vi "Chart[Template].TestLauncher.vi"() -> ()   [LabVIEW 2018, in "DisplayWaveform.lvlib" / "DisplayWaveforms.lvclass"]
doc: "JKI State Machine Objects (SMO) 1.0.0.5\nJKI - JKI\nCopyright (c) 2016, JKI"
uses:
  DisplayWaveforms.lvclass
  <vilib>/JKI/JKI SMO/SMO/SMO.lvclass
  <vilib>/JKI/JKI SMO/SMO.UI/SMO.UI.lvclass
  Typedefs/Dependencies--Cluster.ctl
  <vilib>/JKI/JKI SMO/SMO/Typedefs/SMOState --Enum.ctl
  C:/Program Files (x86)/National Instruments/LabVIEW 2020/vi.lib/JKI/JKI SMO/SMO.UI/SMO.UI.lvclass
  C:/Program Files (x86)/National Instruments/LabVIEW 2020/vi.lib/JKI/JKI SMO/SMO/SMO.lvclass
panel:
  in  "Send":bool
  out "error out":errorcluster
  in  "Stop":bool
  # "Chart Test Launcher"
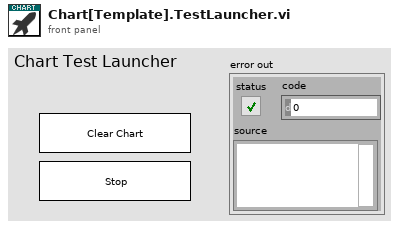
[diagram p1: front panel]
types:
  T1 = typedef "DisplayWaveform.lvlib/DisplayWaveforms.lvclass/Dependencies--Cluster.ctl" = cluster{"New Value":refnum<user-event>}
  T2 = typedef "SMO.lvclass/Public Events.ctl" = cluster{"Error":refnum<user-event>, "State":refnum<user-event>, "Reserve State":refnum<user-event>}
  T3 = typedef "SMO.UI.lvclass/PublicEvents--Cluster.ctl" = cluster{"UI Hidden":refnum<user-event>, "UI State":refnum<user-event>}
  T4 = typedef "DisplayWaveform.lvlib/DisplayWaveforms.lvclass/PublicEvents--Cluster.ctl" = cluster{"Chart Cleared":refnum<user-event>, "Chart Exported":refnum<user-event>, "ChartParams Set":refnum<user-event>}
  T5 = typedef "SMO.lvclass/SMOState --Enum.ctl" = enum16{"unknown", "Created", "Started", "Stopped"}
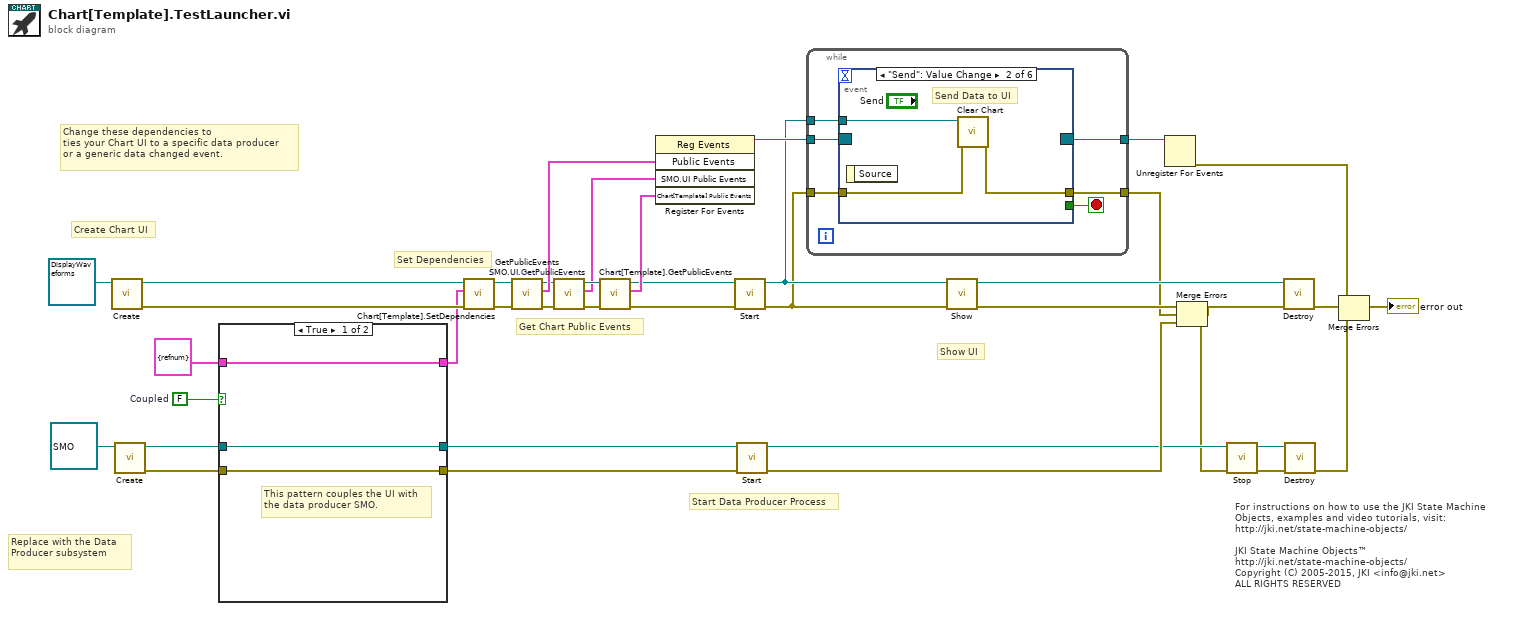
[diagram p0: block diagram]
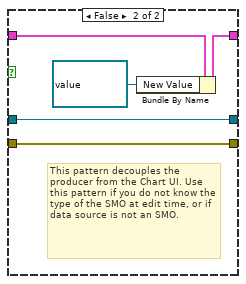
[diagram p2: hidden frame]
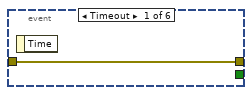
[diagram p3: hidden frame]
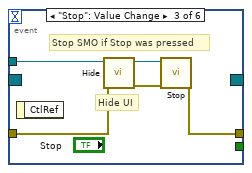
[diagram p4: hidden frame]
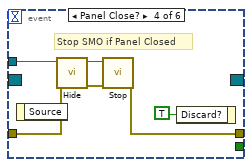
[diagram p5: hidden frame]
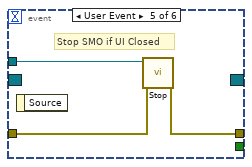
[diagram p6: hidden frame]
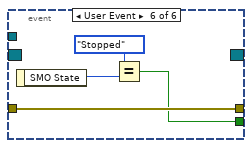
[diagram p7: hidden frame]
diagram:
  w22 = FALSE  # Coupled
  # "Start Data Producer Process"
  # "Set Dependencies"
  # "Create Chart UI"
  # "Replace with the Data Producer subsystem"
  # "Change these dependencies to\nties your Chart UI to a specific data producer\nor a generic data changed event."
  # "Show UI"
  # "For instructions on how to use the JKI State Machine Objects, examples and video tutorials, visit:\nhttp://jki.net/state-machine-objects/\n\nJKI State Machine Objects™\nhttp://jki.net/state-machine-objects/\nCopyright (C) 2005-2015, JKI <info@jki.net>\nALL RIGHTS RESERVED"
  # "Get Chart Public Events"
  n1 = call <vilib>:"Create.vi"("SMO"=refnum<class "DisplayWaveforms.lvclass"> refnum ("Chart[Template]")) -> ("error out"=w31:errorcluster, "SMO out"=w32:refnum<class "DisplayWaveforms.lvclass">)  [unwired: 8 in, 1 out]
  n2 = call <vilib>:"Create.vi"("SMO"=refnum<class "SMO.lvclass"> refnum) -> ("error out"=w18:errorcluster, "SMO out"=w21:refnum<class "SMO.lvclass">)  [unwired: 8 in, 1 out]
  n3 = case shown="True" w22 {
    tunnel: T1 {"New Value"=refnum} ("Dependencies") -> [w39 w46]
    tunnel: [w39 w45] -> w23
    tunnel: w21 -> [w40 w44]
    tunnel: [w40 w44] -> w20
    tunnel: [w41 w43] -> w19
    tunnel: w18 -> [w41 w43]
    frame True {
      # "This pattern couples the UI with\nthe data producer SMO."
    }
    frame False {
      # "This pattern decouples the producer from the Chart UI. Use this pattern if you do not know the type of the SMO at edit time, or if data source is not an SMO."
      n4 = Bundle By Name(cluster=w46, "New Value"=refnum<user-event> refnum) -> (w45:T1)
    }
  }
  n5 = call "Chart[Template].SetDependencies.vi"("error in (no error)"=w31, "Dependencies"=w23, "DisplayWaveforms"=w32) -> ("error out"=w5:errorcluster, "DisplayWaveforms out"=w17:refnum<class "DisplayWaveforms.lvclass">)  [unwired: 7 in]
  n6 = call <vilib>:"GetPublicEvents.vi"("error in (no error)"=w5, "SMO"=w17) -> ("error out"=w12:errorcluster, "Public Events"=w16:T2, "SMO out"=w14:refnum<class "DisplayWaveforms.lvclass">)  [unwired: 7 in]
  n7 = call <vilib>:"SMO.UI.GetPublicEvents.vi"("error in (no error)"=w12, "SMO.UI"=w14) -> ("error out"=w11:errorcluster, "SMO.UI Public Events"=w10:T3, "SMO.UI out"=w13:refnum<class "DisplayWaveforms.lvclass">)  [unwired: 7 in]
  n8 = call "Chart[Template].GetPublicEvents.vi"("error in (no error)"=w11, "DisplayWaveforms"=w13) -> ("error out"=w6:errorcluster, "Chart[Template] Public Events"=w15:T4, "DisplayWaveforms out"=w7:refnum<class "DisplayWaveforms.lvclass">)  [unwired: 7 in]
  n9 = register-events(w16, w10, w15) -> (reference out=w9:refnum<event-registration>)  [unwired: 2 in, 1 out]
  n10 = call <vilib>:"Start.vi"("error in (no error)"=w6, "SMO"=w7) -> ("error out"=w2:errorcluster, "SMO out"=w8:refnum<class "DisplayWaveforms.lvclass">)  [unwired: 8 in]
  n11 = call <vilib>:"Start.vi"("error in (no error)"=w19, "SMO"=w20) -> ("error out"=w29:errorcluster, "SMO out"=w28:refnum<class "SMO.lvclass">)  [unwired: 8 in]
  n12 = while {
    tunnel: w9 -> [w51]
    tunnel: [w50] -> w38
    tunnel: w8 -> [w49]
    tunnel: w2 -> [w48]
    tunnel: [w47] -> w1
    stop <- w52 stop-if-true
    n13 = event shown="[1] \"Send\": Value Change" {
      selector: w51 -> [_ _ _ _ _ _]
      dyn-events: [_ _ _ _ _ _] -> w50
      timeout: _ -> [_ _ _ _ _ _]
      tunnel: [_ _ _ _ _ w71] -> w52
      tunnel: w49 -> [_ w56 w60 w65 w69 _]
      tunnel: [w53 w54 w61 w67 w70 w74] -> w47
      tunnel: w48 -> [w53 w55 w58 w63 w68 w74]
      event Timeout {
        n14 = event-data() -> ()  [unwired: 1 in, 1 out]
      }
      event "Send": Value Change {
        # "Send Data to UI"
        n15 = event-data() -> ()  [unwired: 1 in, 1 out]
        n16 = call "Clear Chart.vi"("error in (no error)"=w55, "DisplayWaveforms"=w56) -> ("error out"=w54:errorcluster)  [unwired: 8 in, 1 out]
      }
      event "Stop": Value Change {
        # "Hide UI"
        # "Stop SMO if Stop was pressed"
        n17 = event-data() -> ()  [unwired: 1 in, 1 out]
        n18 = call <vilib>:"Hide.vi"("error in (no error)"=w58, "SMO.UI"=w60) -> ("error out"=w57:errorcluster, "SMO.UI out"=w59:refnum<class "DisplayWaveforms.lvclass">)  [unwired: 8 in]
        n19 = call <vilib>:"Stop.vi"("error in (no error)"=w57, "SMO"=w59) -> ("error out"=w61:errorcluster)  [unwired: 8 in, 1 out]
      }
      event Panel Close? {
        # "Stop SMO if Panel Closed"
        n20 = event-data() -> ()  [unwired: 1 in, 1 out]
        n21 = call <vilib>:"Hide.vi"("error in (no error)"=w63, "SMO.UI"=w65) -> ("error out"=w62:errorcluster, "SMO.UI out"=w64:refnum<class "DisplayWaveforms.lvclass">)  [unwired: 8 in]
        n22 = call <vilib>:"Stop.vi"("error in (no error)"=w62, "SMO"=w64) -> ("error out"=w67:errorcluster)  [unwired: 8 in, 1 out]
        n23 = event-data("Discard?"=TRUE ("OK")) -> ()  [unwired: 1 in, 1 out]
      }
      event User Event {
        # "Stop SMO if UI Closed"
        n24 = event-data() -> ()  [unwired: 1 in, 1 out]
        n25 = call <vilib>:"Stop.vi"("error in (no error)"=w68, "SMO"=w69) -> ("error out"=w70:errorcluster)  [unwired: 8 in, 1 out]
      }
      event User Event {
        n26 = event-data() -> ("SMO State"=w73:T5)  [unwired: 1 in]
        n27 = Equal?(x=SMOState_--Enum."Stopped", y=w73) -> (x = y?=w71:bool)
      }
    }
  }
  n28 = call <vilib>:"Show.vi"("error in (no error)"=w2, "SMO.UI"=w8) -> ("error out"=w33:errorcluster, "SMO.UI out"=w4:refnum<class "DisplayWaveforms.lvclass">)  [unwired: 8 in]
  n29 = Unregister For Events(event registration refnum=w38) -> (error out=w37:errorcluster)  [unwired: 1 in]
  n30 = Merge Errors(w33, w1, w29) -> (w3:errorcluster)
  n31 = call <vilib>:"Stop.vi"("error in (no error)"=w3, "SMO"=w28) -> ("error out"=w27:errorcluster, "SMO out"=w26:refnum<class "SMO.lvclass">)  [unwired: 8 in]
  n32 = call <vilib>:"Destroy.vi"("error in (no error)"=w3, "SMO"=w4) -> ("error out"=w35:errorcluster)  [unwired: 9 in]
  n33 = call <vilib>:"Destroy.vi"("error in (no error)"=w27, "SMO"=w26) -> ("error out"=w25:errorcluster)  [unwired: 9 in]
  n34 = Merge Errors(w37, w35, w25) -> (→"error out":errorcluster)
